vi "(SubVI) Darg Force Calculation_YCC.vi"(6 "Temperature (C)":dbl, 7 "Velocity (um/s)":dbl, 8 "Volumn of glycerol":dbl, 9 "Volumn of water":dbl, 10 "bead height (um)":dbl=1.0, 11 "bead radius (um)":dbl=0.515) -> (1 "Viscosity of mix (cP)":dbl, 2 "Faxen's law of friction coefficient (pN/(um/s))":dbl, 3 "Drag Force (pN)":dbl)   [LabVIEW 2014]
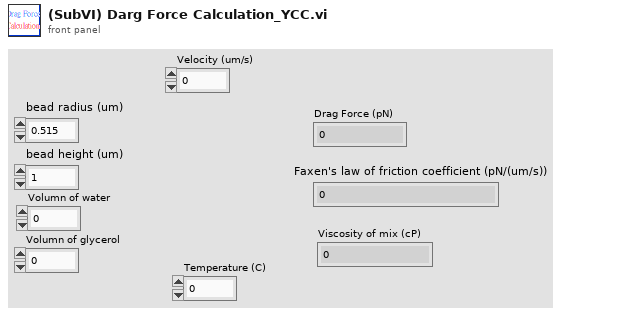
[diagram p1: front panel]
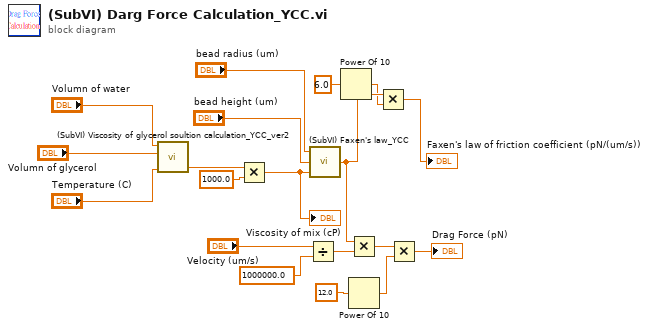
[diagram p0: block diagram]
diagram:
  n1 = call "(SubVI) Viscosity of glycerol soultion calculation_YCC_ver2.vi"("Volumn of water"="Volumn of water", "Volumn of glycerol"="Volumn of glycerol", "Temperature (C)"="Temperature (C)") -> ("Viscosity of mix (Pa*s)"=w17:dbl)  [unwired: 4 in, 1 out]
  n2 = Multiply(x=w17, y=1000.0) -> (x*y=w15:dbl)
  "Viscosity of mix (cP)" <- w15
  n3 = Divide(x="Velocity (um/s)", y=1000000.0) -> (x/y=w9:dbl)
  n4 = call "(SubVI) Faxen's law_YCC.vi"("viscosity (cP)"=w15, "bead height (um)"="bead height (um)", "bead radius (um)"="bead radius (um)") -> ("Faxen's law of friction coefficient (N/(m/s))"=w4:dbl)  [unwired: 2 in]
  n5 = Power Of 10(x=6.0) -> (10^x=w2:dbl)
  n6 = Multiply(x=w4, y=w9) -> (x*y=w8:dbl)
  n7 = Power Of 10(x=12.0) -> (10^x=w6:dbl)
  n8 = Multiply(x=w4, y=w2) -> (x*y=→"Faxen's law of friction coefficient (pN/(um/s))":dbl)
  n9 = Multiply(x=w8, y=w6) -> (x*y=→"Drag Force (pN)":dbl)
